vi "Set Test File Version.vi"(7 "Unique ID":string, 8 "error in (no error)":errorcluster, 10 "Test File Version":string, 11 "Test Executive in":refnum<class "Test Executive.lvclass">) -> (0 "error out":errorcluster, 3 "Test Executive out":refnum<class "Test Executive.lvclass">)   [LabVIEW 2020, in "Test Executive.lvlib" / "Test Executive.lvclass"]
uses:
  <vilib>/gpm_packages/@cs/test-executive/Source/Test Executive/TestExecutive/Test Executive.lvclass
  <vilib>/gpm_packages/@cs/test-executive/Source/Test Executive/TestExecutive/Test Executive.lvclass/Test Executive.ctl
  <vilib>/gpm_packages/@cs/linked-list/Source/Linked List/Linked List Ref/Linked List Ref.lvclass
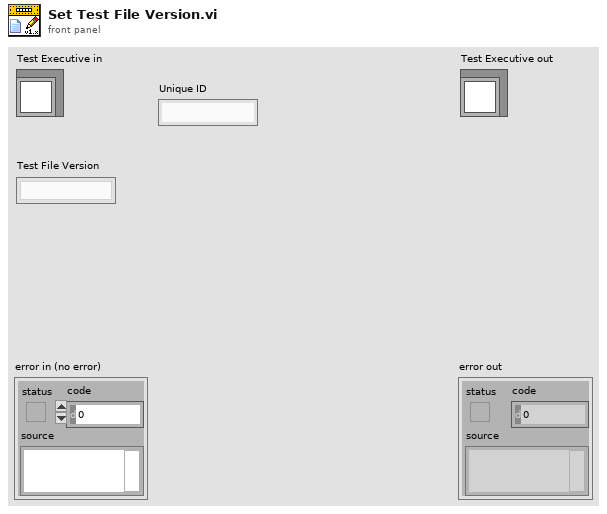
[diagram p1: front panel]
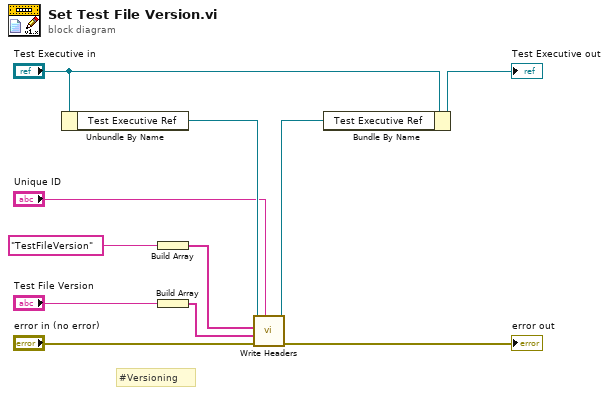
[diagram p0: block diagram]
diagram:
  # "#Versioning"
  n1 = Unbundle By Name("Test Executive in") -> ("Test Executive Ref"=w11:refnum<data-value>)
  n2 = Build Array("TestFileVersion" ("String")) -> (w3:string[])
  n3 = Build Array("Test File Version") -> (w1:string[])
  n4 = call <vilib>:"Write Headers.vi"("Linked List ID"="Unique ID", "error in (no error)"="error in (no error)", "Header Values"=w1, "Header Names"=w3, "Linked List Ref"=w11) -> ("error out"=→"error out":errorcluster, "Linked List Ref out"=w5:refnum<data-value>)  [unwired: 5 in]
  n5 = Bundle By Name(cluster="Test Executive in", "Test Executive Ref"=w5) -> (→"Test Executive out":refnum<class "Test Executive.lvclass">)
